vi "Actor Core.vi"(8 "error in":errorcluster, 11 "SolarSystems M266 Old in":refnum<class "SolarSystems M266 Old.lvclass">) -> (0 "error out":errorcluster, 3 "Actor out":refnum<class "Actor.lvclass">)   [LabVIEW 2014, in "SolarSystems M266 Old.lvclass"]
doc: "(<B>Filename</B>: Actor Framework.lvlib:Actor.lvclass:Actor Core.vi)\n\nReceives messages to the actor, reacts to them, and initiates any error handling that may shut the actor down.\n\nDescendant classes may override this VI to append parallel tasks for the actor to complete while it handles messages. Overrides use the Call Parent Method node."
uses:
  SolarSystems M266 Old.lvclass
  Framework/Hardware/ParameterDevice/ParameterDevice.lvclass
  Framework/Interfaces/Viewable Actor/Viewable Actor.lvclass
  Framework/Interfaces/Observable Actor/Observable Actor.lvclass
  <vilib>/ActorFramework/Actor/Actor.lvclass
  Framework/Hardware/Device/Device Messages/Connect Msg/Connect Msg.lvclass
panel:
  out "Stop":bool=TRUE
  out "Error":string
  in  "Select shutter state":u32(ring) items=["Open", "Close"]
  in  "Set shutter state":bool
  in  "Select filter":i32(ring) items=["Filter1", "Filter2", "Filter3", "Filter4", "Filter5", "Filter6", "Filter7", "Filter8"]
  in  "Set filter":bool
  in  "Select mirror":i32(ring) items=["Axial port", "Lateral port"]
  in  "Set mirror":bool
  in  "New slit width":dbl format="%.2f"
  in  "Reset 2":bool
  in  "Set slit width":bool
  in  "New WL":dbl format="%.2f"
  in  "Reset":bool caption="bReset"
  in  "Set new WL":bool caption="Boolean"
  out "Cur WL":dbl format="%.2f"
  out "Slit width":dbl format="%.2f"
  out "Cur. mirror":u32(ring) items=["Axial port", "Lateral port"]
  out "Cur. filter":i32(ring) items=["Filter1", "Filter2", "Filter3", "Filter4", "Filter5", "Filter6", "Filter7", "Filter8"]
  out "Cur. state":i32(ring) items=["Unknown", "Open", "Close"]
  out "Dispersion":dbl format="%.4f"
  in  "Select slit":u32(ring) items=["Entrance Slit", "Exit Slit"]
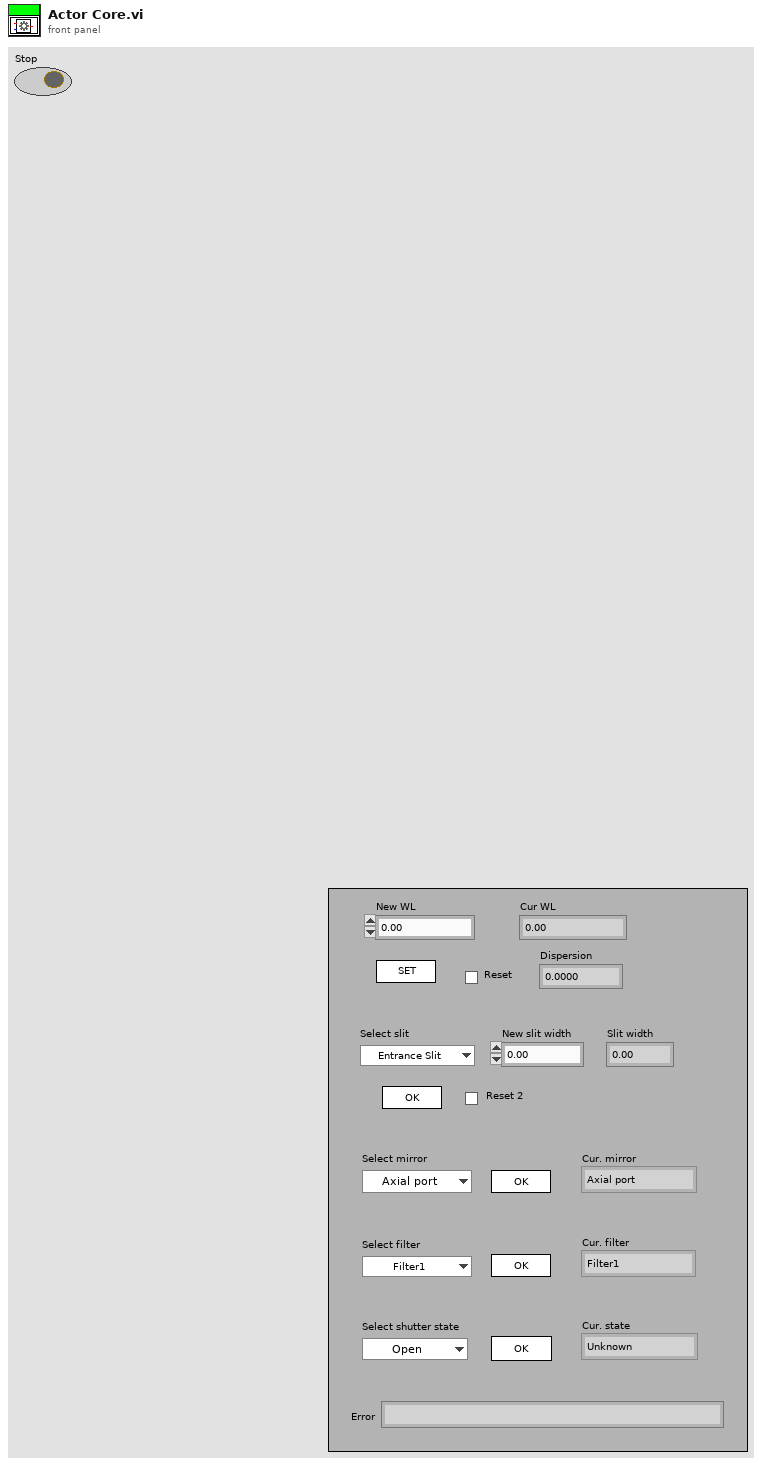
[diagram p1: front panel]
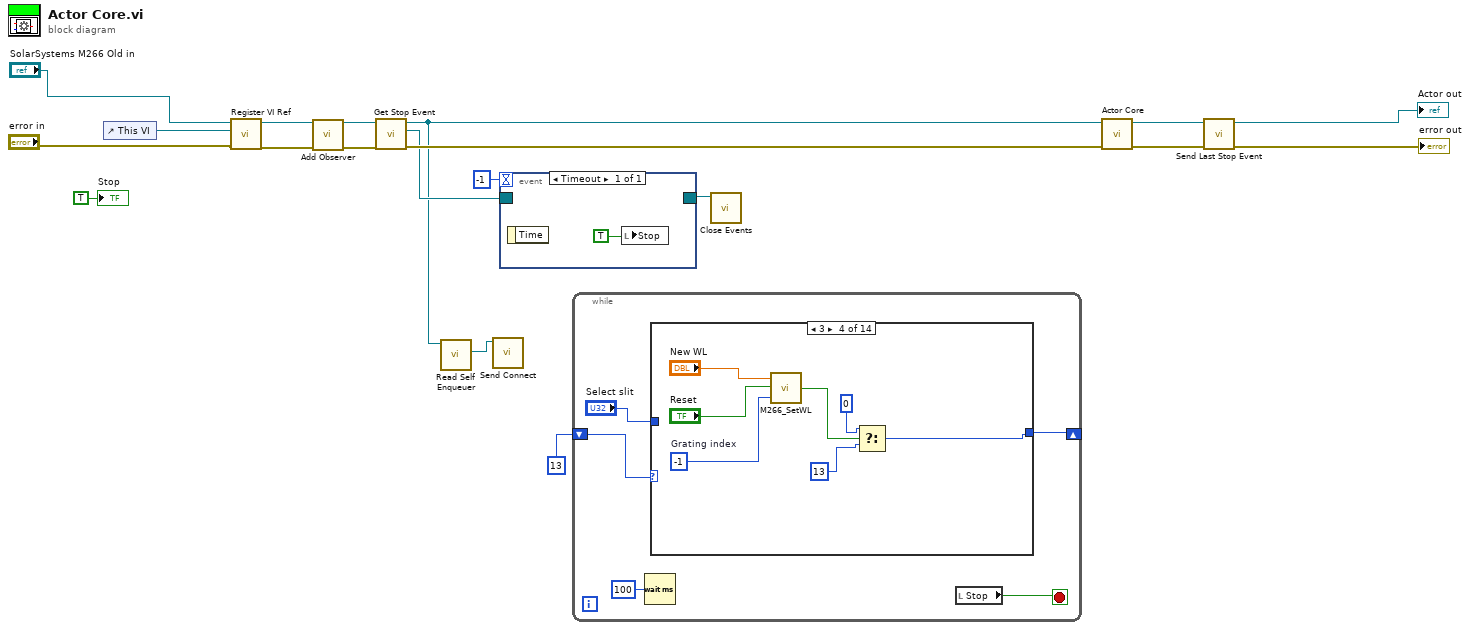
[diagram p0: block diagram]
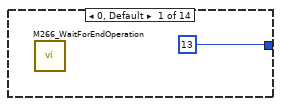
[diagram p2: hidden frame]
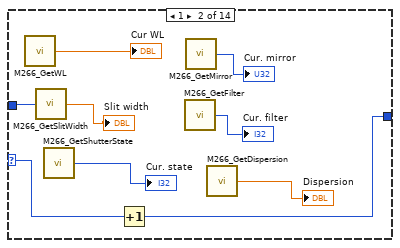
[diagram p3: hidden frame]
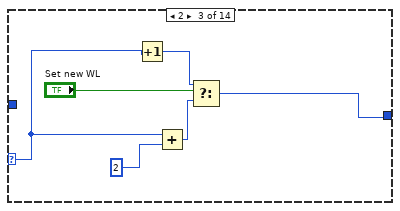
[diagram p4: hidden frame]
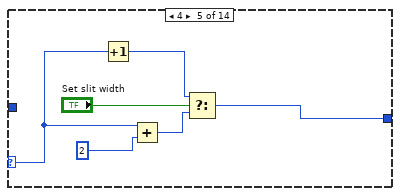
[diagram p5: hidden frame]
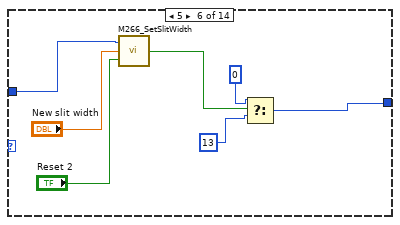
[diagram p6: hidden frame]
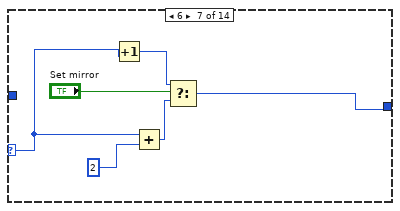
[diagram p7: hidden frame]
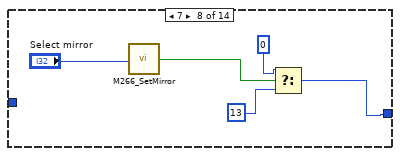
[diagram p8: hidden frame]
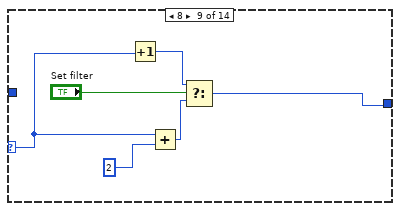
[diagram p9: hidden frame]
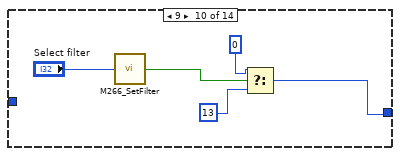
[diagram p10: hidden frame]
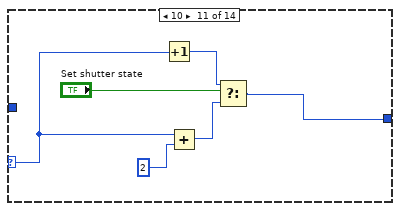
[diagram p11: hidden frame]
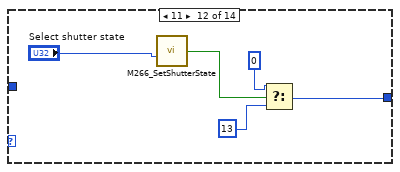
[diagram p12: hidden frame]
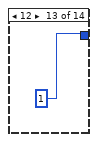
[diagram p13: hidden frame]
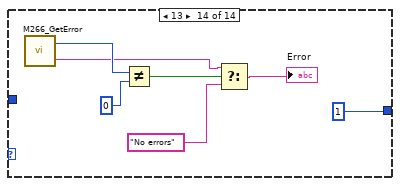
[diagram p14: hidden frame]
diagram:
  n1 = control-ref of="This VI"() -> (w12:refnum<vi>)
  n2 = call "Register VI Ref.vi"("error in (no error)"="error in", "VI ref"=w12, "Viewable Actor in"="SolarSystems M266 Old in") -> ("error out"=w14:errorcluster, "Viewable Actor out"=w13:refnum<class "SolarSystems M266 Old.lvclass">)  [unwired: 7 in]
  n3 = call-dynamic "Add Observer.vi"("error in (no error)"=w14, "Observable Actor in"=w13) -> ("error out"=w19:errorcluster, "Observable Actor out"=w18:refnum<class "SolarSystems M266 Old.lvclass">)  [unwired: 7 in, 1 out]
  n4 = call-dynamic "Get Stop Event.vi"("error in (no error)"=w19, "Observable Actor in"=w18) -> ("error out"=w17:errorcluster, "Events"=w10:refnum<event-registration>, "Observable Actor out"=w7:refnum<class "SolarSystems M266 Old.lvclass">)  [unwired: 7 in]
  n5 = call <vilib>:"Read Self Enqueuer.vi"("Actor"=w7) -> ("Self Enqueuer"=w6:refnum<class "Message Enqueuer.lvclass">)  [unwired: 10 in]
  n6 = call "Send Connect.vi"("Message Enqueuer"=w6) -> ()  [unwired: 9 in, 2 out]
  n7 = event shown="[0] Timeout" {
    selector: w10 -> [_]
    dyn-events: [_] -> w8
    timeout: -1 ("Numeric") -> [_]
    event Timeout {
      n8 = event-data() -> ()  [unwired: 1 in, 1 out]
      n9 = local write "Stop"(TRUE) -> ()
    }
  }
  n10 = while {
    shift-right: [w24] -> _
    shift-left: 13 -> [w23]
    stop <- w22 stop-if-true
    n11 = Wait (ms)(milliseconds to wait=u32 100) -> ()  [unwired: 1 out]
    n12 = case shown="3" w23 {
      selector: w23 -> [_ w31 w36 _ w49 _ w63 _ w74 _ w87 _ _ _]
      tunnel: "Select slit" -> [_ w33 _ _ _ w55 _ _ _ _ _ _ _ _]
      tunnel: [13 w32 w40 w43 w50 w56 w62 w69 w73 w79 w84 w91 1 1] -> w24
      frame 0, Default {
        n13 = call "M266_WaitForEndOperation.vi"() -> ()  [unwired: 1 out]
      }
      frame 1 {
        n14 = call "M266_GetWL.vi"() -> ("Current WL"=→"Cur WL":dbl)
        n15 = call "M266_GetSlitWidth.vi"("Select slit"=w33) -> ("Slit width"=→"Slit width":dbl)
        n16 = call "M266_GetShutterState.vi"() -> ("Shutter state"=→"Cur. state":i32)
        n17 = Increment(x=w31) -> (x+1=w32:i32)
        n18 = call "M266_GetFilter.vi"() -> ("Filter"=→"Cur. filter":i32)
        n19 = call "M266_GetMirror.vi"() -> ("Mirror position"=→"Cur. mirror":i32)
        n20 = call "M266_GetDispersion.vi"() -> ("Dispersion"=→"Dispersion":dbl)
      }
      frame 2 {
        n21 = Increment(x=w36) -> (x+1=w39:i32)
        n22 = Add(x=w36, y=2) -> (x+y=w37:i32)
        n23 = Select(t=w39, s="Set new WL", f=w37) -> (s? t:f=w40:i32)
      }
      frame 3 {
        w47 = -1  # Grating index
        n24 = call "M266_SetWL.vi"("Grating index"=w47, "Reset"="Reset", "WL"="New WL") -> ("Result"=w46:bool)
        n25 = Select(t=0, s=w46, f=13) -> (s? t:f=w43:i32)
      }
      frame 4 {
        n26 = Increment(x=w49) -> (x+1=w53:i32)
        n27 = Add(x=w49, y=2) -> (x+y=w52:i32)
        n28 = Select(t=w53, s="Set slit width", f=w52) -> (s? t:f=w50:i32)
      }
      frame 5 {
        n29 = call "M266_SetSlitWidth.vi"("Reset"="Reset 2", "Slit width"="New slit width", "Select slit"=w55) -> ("Result"=w58:bool)
        n30 = Select(t=0, s=w58, f=13) -> (s? t:f=w56:i32)
      }
      frame 6 {
        n31 = Increment(x=w63) -> (x+1=w67:i32)
        n32 = Add(x=w63, y=2) -> (x+y=w65:i32)
        n33 = Select(t=w67, s="Set mirror", f=w65) -> (s? t:f=w62:i32)
      }
      frame 7 {
        n34 = call "M266_SetMirror.vi"("Select mirror"="Select mirror") -> ("Result"=w70:bool)
        n35 = Select(t=0, s=w70, f=13) -> (s? t:f=w69:i32)
      }
      frame 8 {
        n36 = Increment(x=w74) -> (x+1=w78:i32)
        n37 = Add(x=w74, y=2) -> (x+y=w76:i32)
        n38 = Select(t=w78, s="Set filter", f=w76) -> (s? t:f=w73:i32)
      }
      frame 9 {
        n39 = call "M266_SetFilter.vi"("Select filter"="Select filter") -> ("Result"=w80:bool)
        n40 = Select(t=0, s=w80, f=13) -> (s? t:f=w79:i32)
      }
      frame 10 {
        n41 = Increment(x=w87) -> (x+1=w89:i32)
        n42 = Add(x=w87, y=2) -> (x+y=w85:i32)
        n43 = Select(t=w89, s="Set shutter state", f=w85) -> (s? t:f=w84:i32)
      }
      frame 11 {
        n44 = call "M266_SetShutterState.vi"("Select shutter state"="Select shutter state") -> ("Result"=w92:bool)
        n45 = Select(t=0, s=w92, f=13) -> (s? t:f=w91:i32)
      }
      frame 12 {
      }
      frame 13 {
        n46 = call "M266_GetError.vi"() -> ("Error text"=w97:string, "Error code"=w102:u32)
        n47 = Not Equal?(x=w102, y=0) -> (x != y?=w99:bool)
        n48 = Select(t=w97, s=w99, f="No errors") -> (s? t:f=→"Error":string)
      }
    }
    n49 = local read "Stop"() -> (w22:bool)
  }
  n50 = call "Close Events.vi"("events"=w8) -> ()  [unwired: 11 in]
  n51 = call-parent "Actor Core.vi"("error in"=w17, "Actor in"=w7) -> ("error out"=w15:errorcluster, "Actor out"=w16:refnum<class "Actor.lvclass">)  [unwired: 8 in]
  n52 = call "Send Last Stop Event.vi"("error in (no error)"=w15, "Actor in"=w16) -> ("error out"=→"error out":errorcluster, "Actor  out"=→"Actor out":refnum<class "Actor.lvclass">)  [unwired: 8 in]
  "Stop" <- TRUE ("Stop")
